vi "getControlPoint.vi"(0 "reference":refnum<class "StateTransitionEdge.lvclass">, 5 "error in (no error)":errorcluster) -> (14 "reference out":refnum<class "StateTransitionEdge.lvclass">, 15 "point":T1 {"y" format="%.2f"; "x" format="%.2f"}, 19 "error out":errorcluster)   [LabVIEW 2020, in "StateTransitionEdge.lvclass"]
doc: "Point2D getControlPoint()"
uses:
  <resource>/Framework/Providers/Open_GDS/UML/StateTransitionEdge_class/StateTransitionEdge.lvclass
  <resource>/Framework/Providers/Open_GDS/UML/General/Point/Point Point2D.ctl
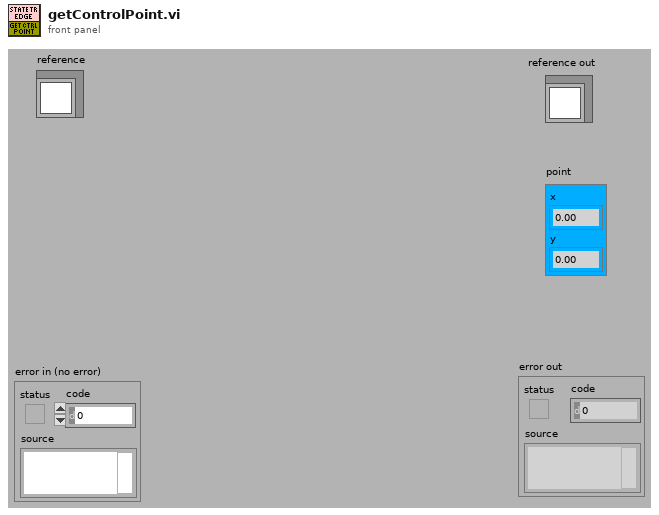
[diagram p1: front panel]
types:
  T1 = typedef "Point Point2D.ctl" = cluster{"x":dbl, "y":dbl}
  T2 = typedef "StateTransitionEdge.lvclass/ObjectAttributes.ctl" = cluster{"angle":dbl}
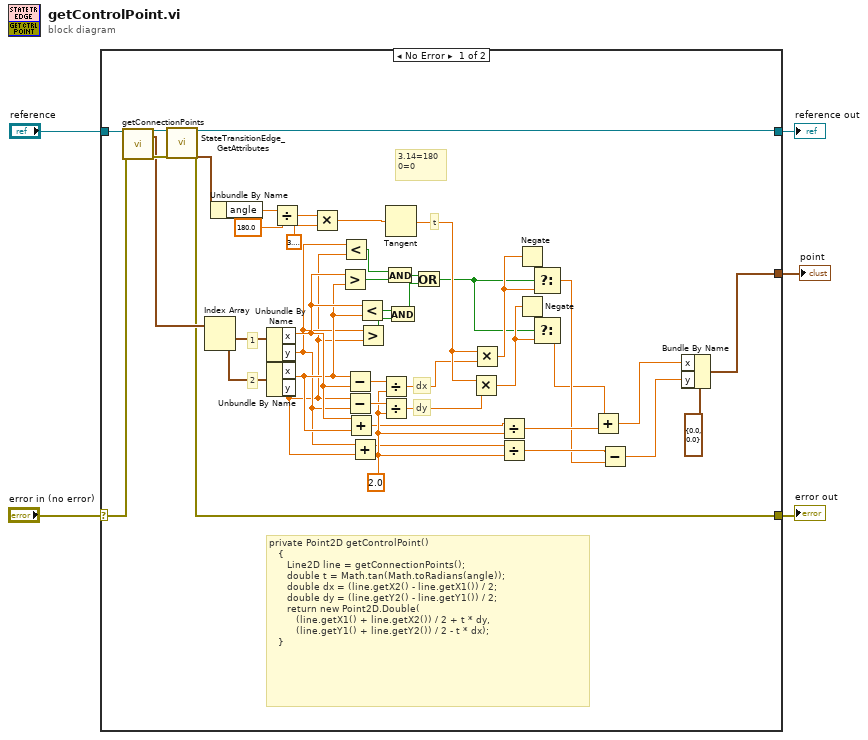
[diagram p0: block diagram]
diagram:
  n1 = case shown="No Error" "error in (no error)" {
    selector: "error in (no error)" -> [w50 w52]
    tunnel: "reference" -> [w51 w53]
    tunnel: [w35 w52] -> w4
    tunnel: [w47 w53] -> w3
    tunnel: [w36 _] -> w1
    frame No Error {
      w34 = 2.0 ("y")
      # "dy"
      # "dx"
      # "t"
      # "2"
      # "1"
      # "3.14=180\n0=0"
      # "private Point2D getControlPoint()\n   {\n      Line2D line = getConnectionPoints();\n      double t = Math.tan(Math.toRadians(angle));\n      double dx = (line.getX2() - line.getX1()) / 2;\n      double dy = (line.getY2() - line.getY1()) / 2;\n      return new Point2D.Double(\n         (line.getX1() + line.getX2()) / 2 + t * dy,\n         (line.getY1() + line.getY2()) / 2 - t * dx);         \n   }"
      n2 = call-dynamic "getConnectionPoints.vi"("reference"=w51, "error in (no error)"=w50) -> ("reference out"=w49:refnum<class "StateTransitionEdge.lvclass">, "line"=w42:T1[], "error out"=w48:errorcluster)  [unwired: 15 in]
      n3 = call <resource>:"StateTransitionEdge_GetAttributes.vi"("reference in"=w49, "error in (no error)"=w48) -> ("reference out"=w47:refnum<class "StateTransitionEdge.lvclass">, "Data"=w6:T2, "error out"=w35:errorcluster)  [unwired: 1 in, 14 out]
      n4 = Index Array(array=w42) -> (element #1=w41:T1, element #2=w40:T1)  [unwired: 2 in]
      n5 = Unbundle By Name(w6) -> ("angle"=w46:dbl)
      n6 = Unbundle By Name(w41) -> ("x"=w13:dbl, "y"=w8:dbl)
      n7 = Unbundle By Name(w40) -> ("x"=w12:dbl, "y"=w7:dbl)
      n8 = Divide(x=w46, y=180.0) -> (x/y=w44:dbl)
      n9 = Multiply(x=w44, y=3.141592653589793) -> (x*y=w24:dbl)
      n10 = Greater?(x=w13, y=w12) -> (0:w14:bool)
      n11 = Less?(x=w8, y=w7) -> (x < y?=w15:bool)
      n12 = Subtract(x=w12, y=w13) -> (x-y=w39:dbl)
      n13 = Subtract(x=w7, y=w8) -> (x-y=w38:dbl)
      n14 = Add(x=w13, y=w12) -> (x+y=w33:dbl)
      n15 = Add(x=w8, y=w7) -> (x+y=w28:dbl)
      n16 = Less?(x=w13, y=w12) -> (x < y?=w11:bool)
      n17 = Greater?(x=w8, y=w7) -> (0:w10:bool)
      n18 = Divide(x=w39, y=w34) -> (x/y=w29:dbl)
      n19 = Divide(x=w38, y=w34) -> (x/y=w31:dbl)
      n20 = And(x=w15, y=w14) -> (x .and. y?=w17:bool)
      n21 = Tangent(1:w24) -> (0:w30:dbl)
      n22 = And(x=w11, y=w10) -> (x .and. y?=w9:bool)
      n23 = Or(x=w17, y=w9) -> (x .or. y?=w16:bool)
      n24 = Multiply(x=w30, y=w31) -> (x*y=w19:dbl)
      n25 = Multiply(x=w30, y=w29) -> (x*y=w21:dbl)
      n26 = Divide(x=w33, y=w34) -> (x/y=w32:dbl)
      n27 = Divide(x=w28, y=w34) -> (x/y=w27:dbl)
      n28 = Negate(x=w21) -> (-x=w23:dbl)
      n29 = Negate(x=w19) -> (-x=w22:dbl)
      n30 = Select(t=w23, s=w16, f=w21) -> (s? t:f=w20:dbl)
      n31 = Select(t=w22, s=w16, f=w19) -> (s? t:f=w18:dbl)
      n32 = Add(x=w18, y=w32) -> (x+y=w26:dbl)
      n33 = Subtract(x=w27, y=w20) -> (x-y=w25:dbl)
      n34 = Bundle By Name(cluster=T1 {"x"=0.0, "y"=0.0} ("point"), "x"=w26, "y"=w25) -> (w36:T1)
    }
    frame Error {
    }
  }
  "reference out" <- w3
  "error out" <- w4
  "point" <- w1
